vi "sub_ofdm_mes_ce.vi"(11 "ZF channel estimates":cdb[](array[numeric])) -> (3 "interpolated mes carrier CE":cdb[](array[numeric]))   [LabVIEW 2014]
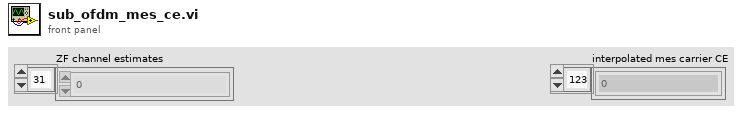
[diagram p1: front panel]
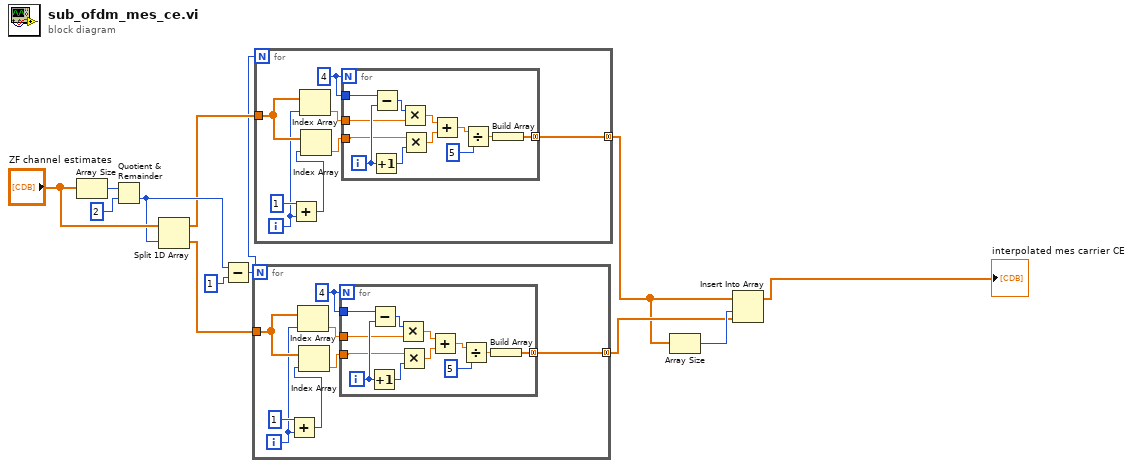
[diagram p0: block diagram]
diagram:
  n1 = Array Size(array="ZF channel estimates") -> (size(s)=w12:i32)
  n2 = Quotient & Remainder(x=w12, y=2) -> (floor(x/y)=w4:i32)  [unwired: 1 out]
  n3 = Split 1D Array(array="ZF channel estimates", index=w4) -> (first subarray=w3:cdb[], second subarray=w9:cdb[])
  n4 = Subtract(x=w4, y=1) -> (x-y=w1:i32)
  n5 = for {
    N: w1 -> [_]
    tunnel: w9 -> [w19]
    tunnel: [w13] -> w5 mode=concatenating
    i -> [w18]
    w16 = 4
    n6 = Add(x=1, y=w18) -> (x+y=w17:i32)
    n7 = Index Array(array=w19, index=w18) -> (element=w15:cdb)
    n8 = Index Array(array=w19, index=w17) -> (element=w14:cdb)
    n9 = for {
      N: w16 -> [_]
      tunnel: w16 -> [w32]
      tunnel: w15 -> [w28]
      tunnel: w14 -> [w27]
      tunnel: [w21] -> w13 mode=concatenating
      i -> [w31]
      n10 = Increment(x=w31) -> (x+1=w29:i32)
      n11 = Subtract(x=w32, y=w31) -> (x-y=w30:i32)
      n12 = Multiply(x=w30, y=w28) -> (x*y=w25:cdb)
      n13 = Multiply(x=w27, y=w29) -> (x*y=w26:cdb)
      n14 = Add(x=w25, y=w26) -> (x+y=w24:cdb)
      n15 = Divide(x=w24, y=5) -> (x/y=w22:cdb)
      n16 = Build Array(w22) -> (w21:cdb[])
    }
  }
  n17 = for {
    N: w1 -> [_]
    tunnel: w3 -> [w39]
    tunnel: [w33] -> w2 mode=concatenating
    i -> [w38]
    w36 = 4
    n18 = Add(x=1, y=w38) -> (x+y=w37:i32)
    n19 = Index Array(array=w39, index=w38) -> (element=w35:cdb)
    n20 = Index Array(array=w39, index=w37) -> (element=w34:cdb)
    n21 = for {
      N: w36 -> [_]
      tunnel: w36 -> [w52]
      tunnel: w35 -> [w48]
      tunnel: w34 -> [w47]
      tunnel: [w41] -> w33 mode=concatenating
      i -> [w51]
      n22 = Increment(x=w51) -> (x+1=w49:i32)
      n23 = Subtract(x=w52, y=w51) -> (x-y=w50:i32)
      n24 = Multiply(x=w50, y=w48) -> (x*y=w45:cdb)
      n25 = Multiply(x=w47, y=w49) -> (x*y=w46:cdb)
      n26 = Add(x=w45, y=w46) -> (x+y=w44:cdb)
      n27 = Divide(x=w44, y=5) -> (x/y=w42:cdb)
      n28 = Build Array(w42) -> (w41:cdb[])
    }
  }
  n29 = Array Size(array=w2) -> (size(s)=w6:i32)
  n30 = Insert Into Array(array=w2, index=w6, new element=w5) -> (→"interpolated mes carrier CE":cdb[])
